vi "Loop.vi"(8 "error in":errorcluster, 10 "UI Queue":refnum<queue>, 11 "Controller Queue":T1) -> (0 "error out":errorcluster)   [LabVIEW 2019, in "Controller.lvlib"]
uses:
  Controller.lvlib
  UI/Update Message.ctl
  UI/Update Command.ctl
  Controller Message Queue.ctl
  Controller Message.ctl
  MDS Command.ctl
  Controller States.ctl
  Serial Info.ctl
  VMode.ctl
  IMode.ctl
  <vilib>/Instr/_visa.llb/VISA Configure Serial Port (Instr).vi
  UI/UI.lvlib
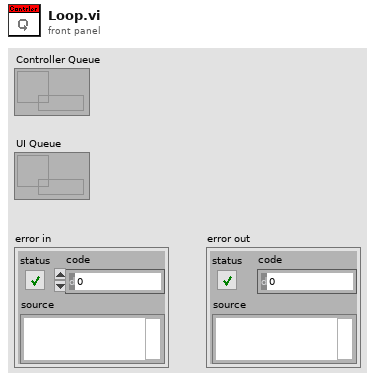
[diagram p1: front panel]
types:
  T1 = typedef "Controller.lvlib/Controller Message Queue.ctl" = refnum<queue>
  T2 = typedef "Controller.lvlib/Controller Message.ctl" = cluster{"MDS Command":T3, "Channel":u8, "Value":variant}
  T3 = typedef "Controller.lvlib/MDS Command.ctl" = enum16{"Idle", "Open", "Set VMode", "Set IMode", "Get Frequency", "Set Frequency", "Get Power", "Set Power (dBm)", "Set Power (%)", "Get Switch", "Switch Channel", "Store", "Wait for Prompt", "Wait for State", "Reset", "Error", "Close", "Stop"}
  T4 = typedef "Controller.lvlib/Controller States.ctl" = cluster{"Resource":refnum<visa-resource-name>}
  T5 = typedef "Controller.lvlib/Serial Info.ctl" = cluster{"Port":refnum<visa-resource-name>, "Baud Rate":u32}
  T6 = typedef "Controller.lvlib/VMode.ctl" = enum8{"5V", "10V"}
  T7 = typedef "Controller.lvlib/IMode.ctl" = enum8{"Internal", "External"}
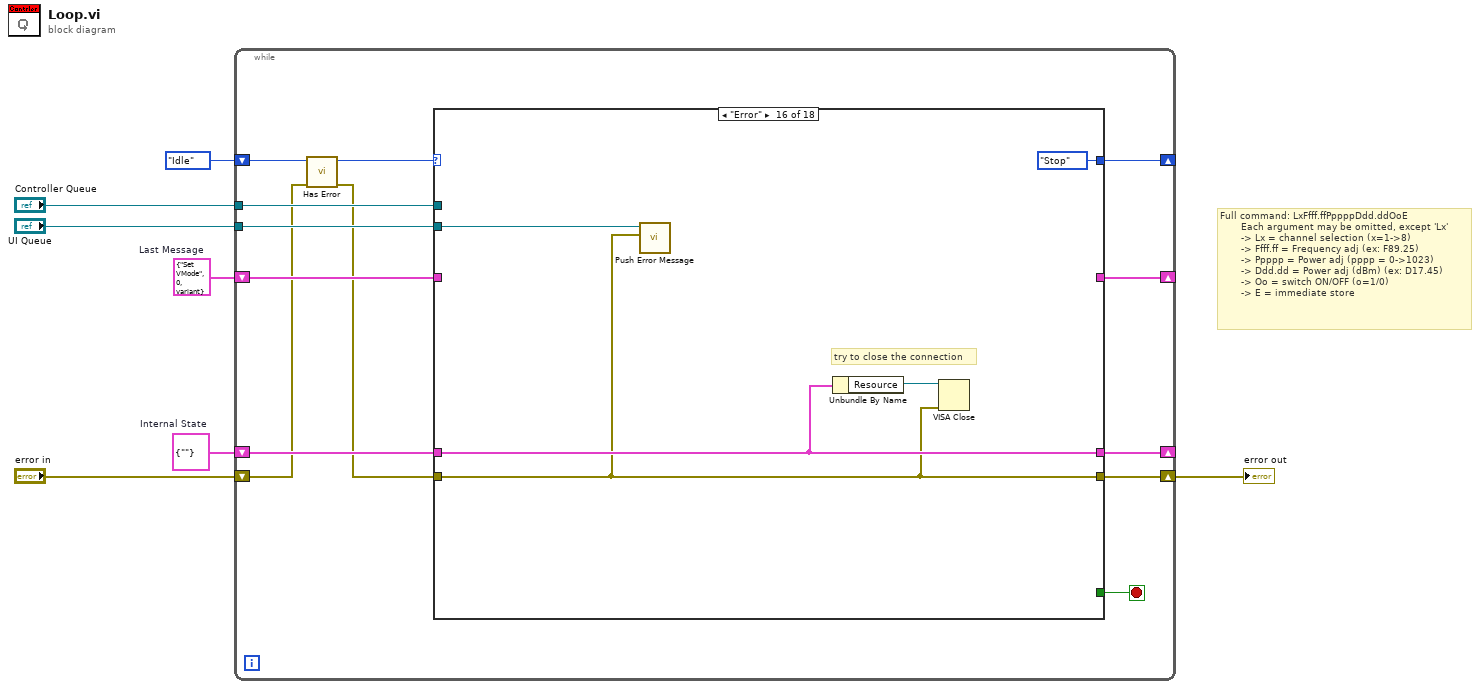
[diagram p0: block diagram]
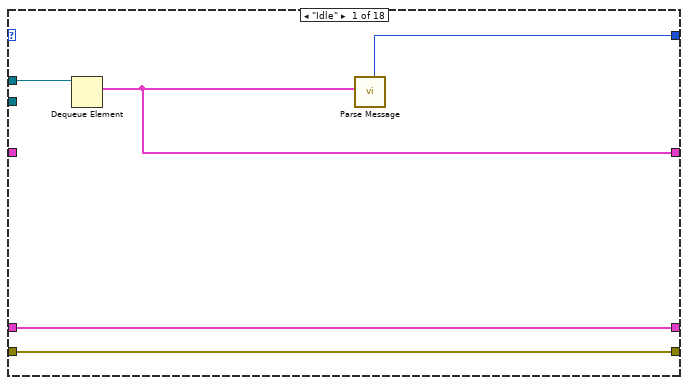
[diagram p2: hidden frame]
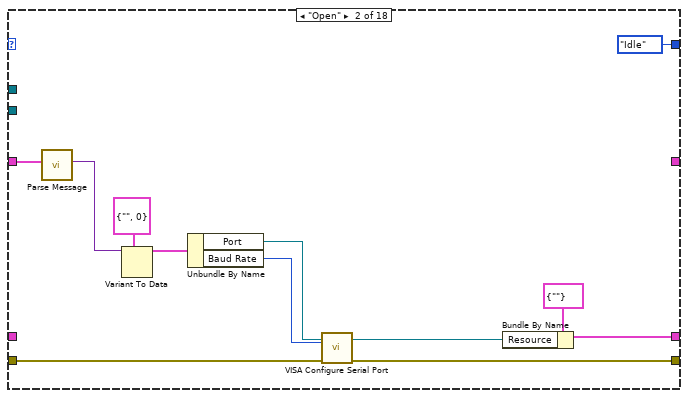
[diagram p3: hidden frame]
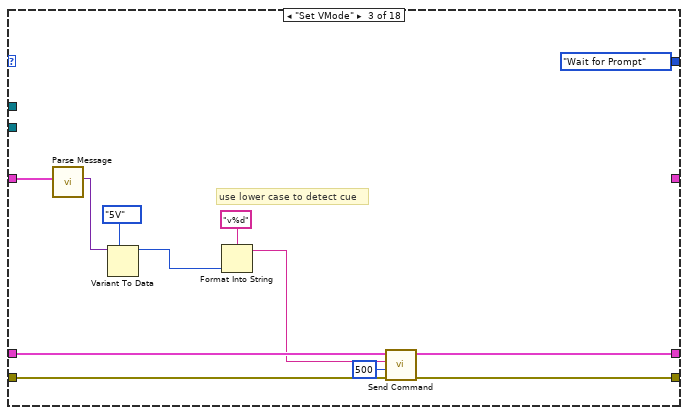
[diagram p4: hidden frame]
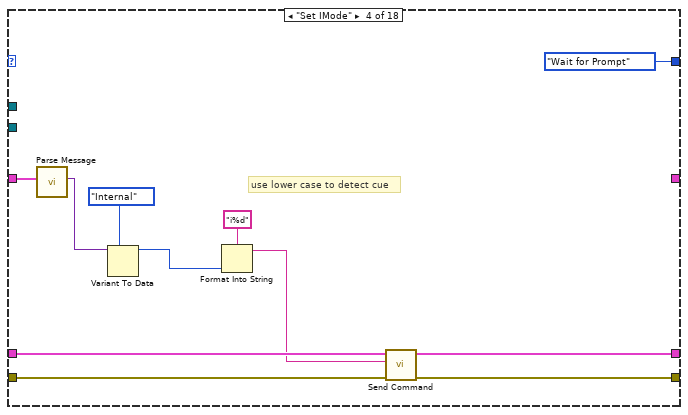
[diagram p5: hidden frame]
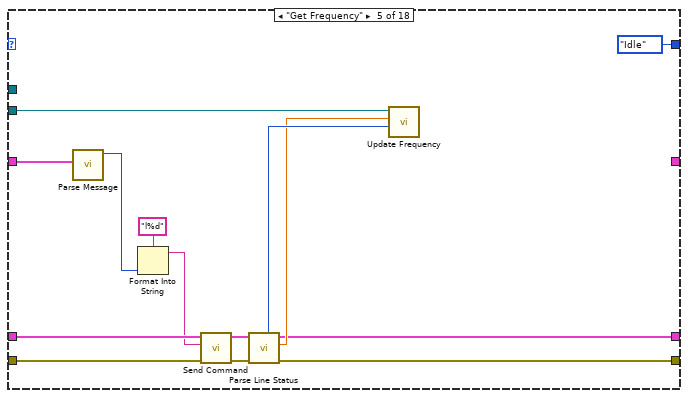
[diagram p6: hidden frame]
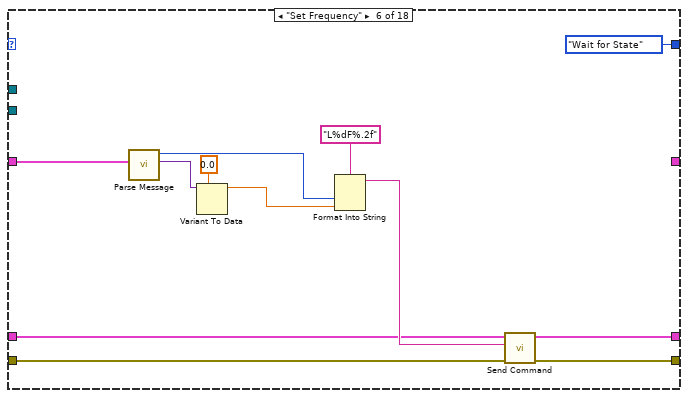
[diagram p7: hidden frame]
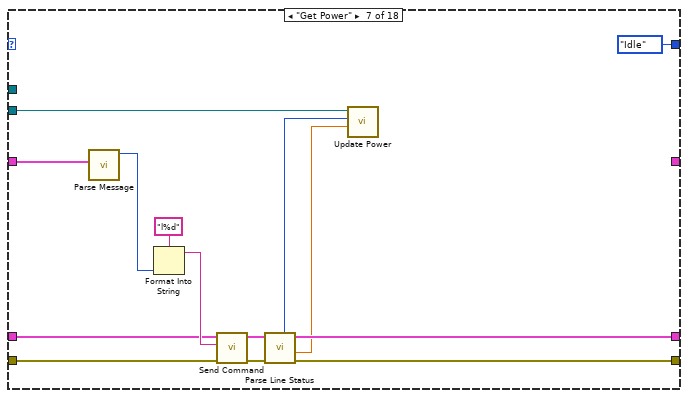
[diagram p8: hidden frame]
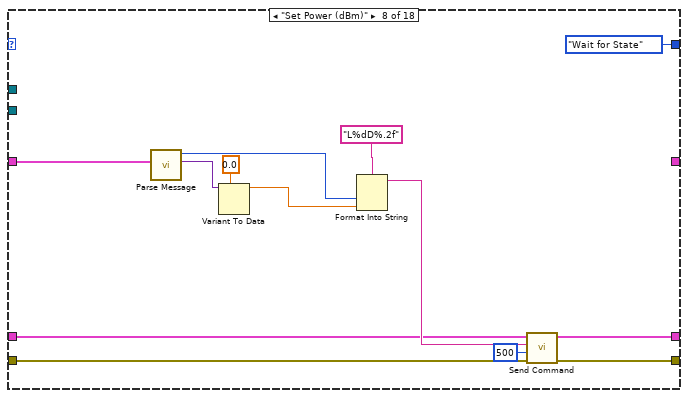
[diagram p9: hidden frame]
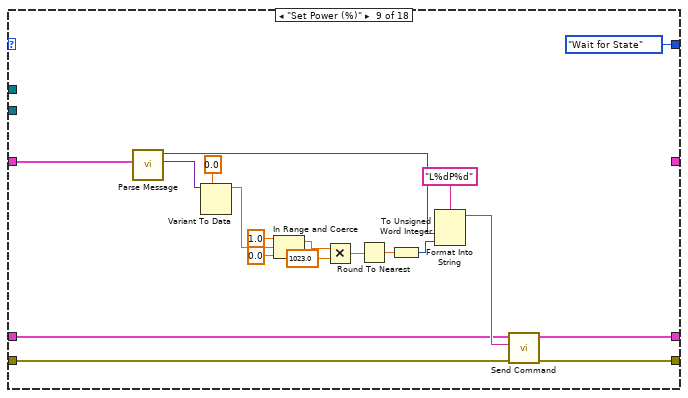
[diagram p10: hidden frame]
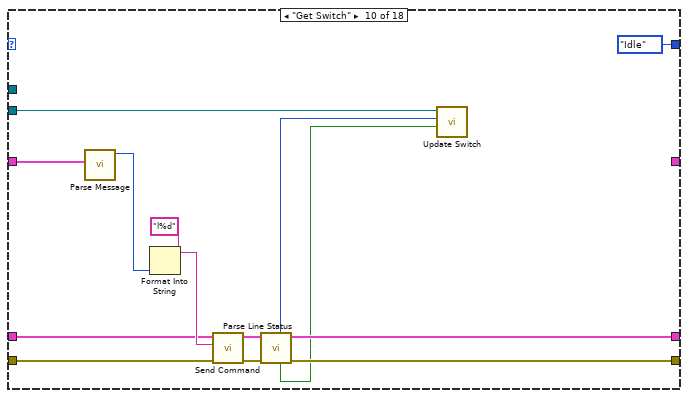
[diagram p11: hidden frame]
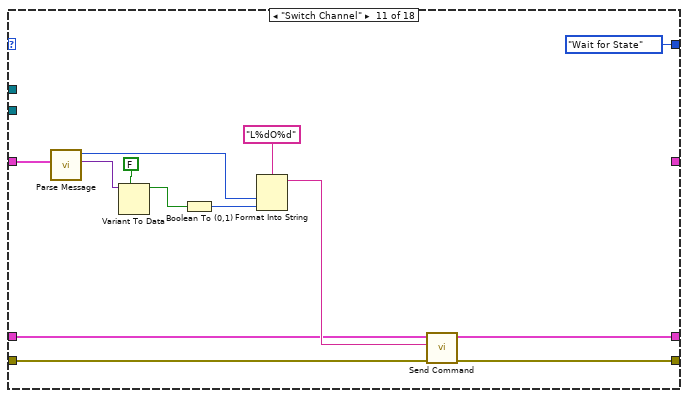
[diagram p12: hidden frame]
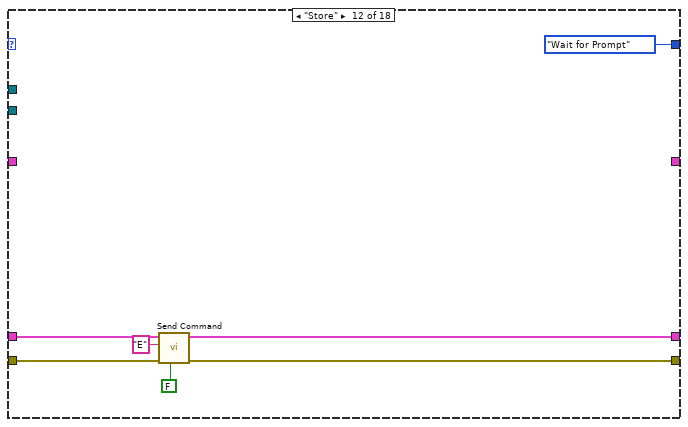
[diagram p13: hidden frame]
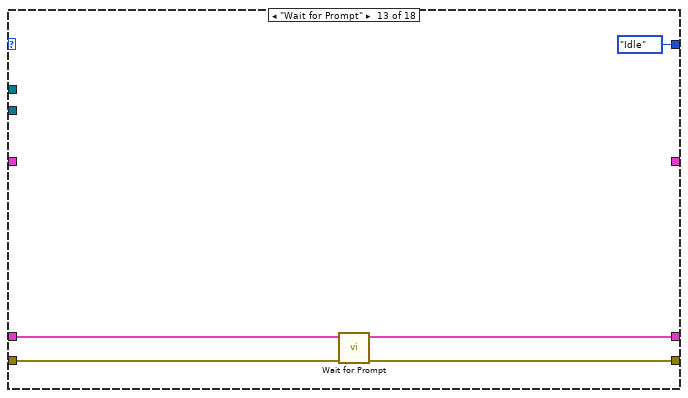
[diagram p14: hidden frame]
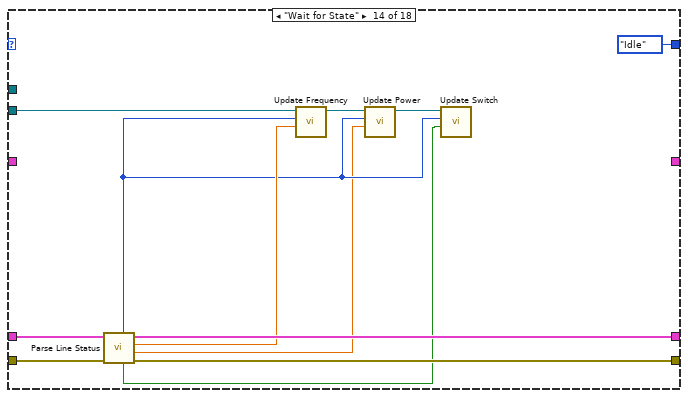
[diagram p15: hidden frame]
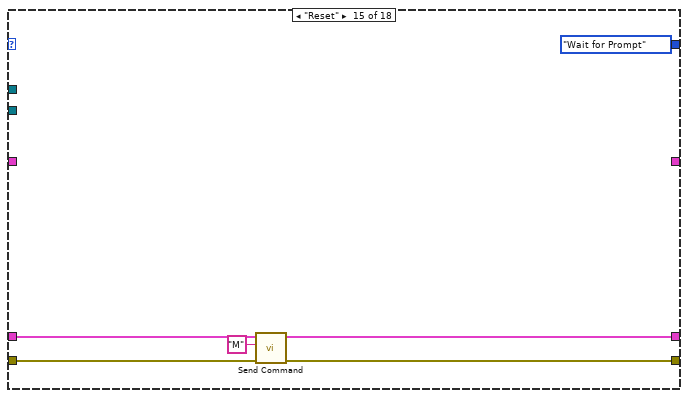
[diagram p16: hidden frame]
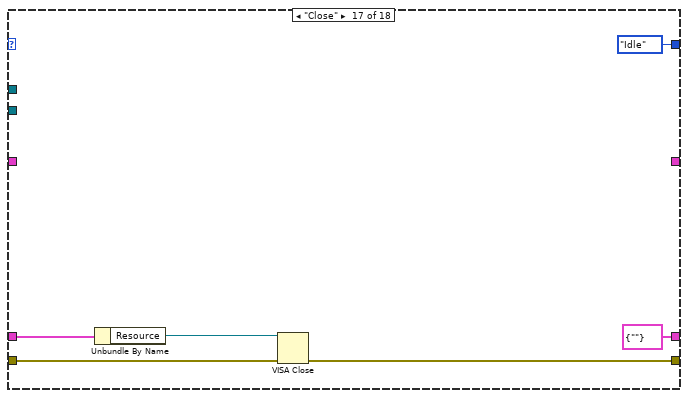
[diagram p17: hidden frame]
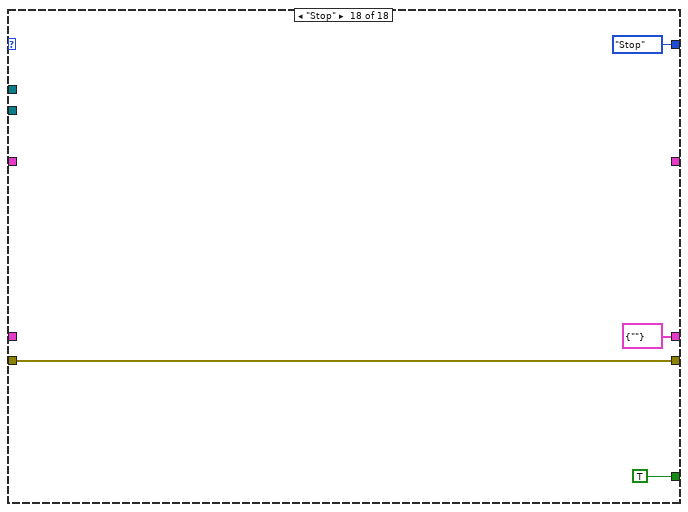
[diagram p18: hidden frame]
diagram:
  w5 = T2 {"MDS Command"=enum."Set VMode", "Channel"=0, "Value"=variant}  # Last Message
  w7 = T4 {"Resource"=""}  # Internal State
  # "Full command: LxFfff.ffPppppDdd.ddOoE\n       Each argument may be omitted, except 'Lx'\n       -> Lx = channel selection (x=1->8)\n       -> Ffff.ff = Frequency adj (ex: F89.25)\n       -> Ppppp = Power adj (pppp = 0->1023)\n       -> Ddd.dd = Power adj (dBm) (ex: D17.45)\n       -> Oo = switch ON/OFF (o=1/0)\n       -> E = immediate store"
  n1 = while {
    tunnel: "Controller Queue" -> [w17]
    shift-right: [w20] -> _
    shift-left: w7 -> [w19]
    shift-right: [w14] -> w4
    shift-left: "error in" -> [w8]
    shift-right: [w15] -> _
    shift-left: w5 -> [w16]
    shift-right: [w12] -> _
    shift-left: MDS_Command."Idle" ("MDS Command") -> [w11]
    tunnel: "UI Queue" -> [w13]
    stop <- w18 stop-if-true
    n2 = call "Has Error.vi"("error in (no error)"=w8, "MDS Command in"=w11) -> ("error out"=w9:errorcluster, "MDS Command out"=w10:T3)  [unwired: 8 in]
    n3 = case shown="\"Error\"" w10 {
      tunnel: [w25 w33 w39 w50 w70 w79 w92 w103 w122 w138 w147 w161 w167 w180 w184 w193 T4 {"Resource"=""} T4 {"Resource"=""}] -> w20
      tunnel: w19 -> [w25 _ w47 w57 w67 w81 w93 w106 w126 w141 w150 w166 w170 w182 w187 w193 w199 _]
      tunnel: w9 -> [w24 w30 w48 w59 w68 w80 w94 w105 w125 w140 w149 w165 w169 w181 w186 w190 w197 w204]
      tunnel: [w24 w29 w38 w58 w71 w78 w91 w104 w123 w139 w148 w160 w168 w179 w185 w190 w196 w204] -> w14
      tunnel: [_ _ _ _ _ _ _ _ _ _ _ _ _ _ _ _ _ TRUE] -> w18
      tunnel: w17 -> [w23 _ _ _ _ _ _ _ _ _ _ _ _ _ _ _ _ _]
      tunnel: w16 -> [_ w27 w41 w52 w63 w77 w90 w102 w124 w136 w158 _ _ _ _ _ _ _]
      tunnel: [w22 _ _ _ _ _ _ _ _ _ _ _ _ _ _ _ _ _] -> w15
      tunnel: [w21 MDS_Command."Idle" ("MDS Command") MDS_Command."Wait for Prompt" ("MDS Command") MDS_Command."Wait for Prompt" ("MDS Command") MDS_Command."Idle" ("MDS Command") MDS_Command."Wait for State" ("MDS Command") MDS_Command."Idle" ("MDS Command") MDS_Command."Wait for State" ("MDS Command") MDS_Command."Wait for State" ("MDS Command") MDS_Command."Idle" ("MDS Command") MDS_Command."Wait for State" ("MDS Command") MDS_Command."Wait for Prompt" ("MDS Command") MDS_Command."Idle" ("MDS Command") MDS_Command."Idle" ("MDS Command") MDS_Command."Wait for Prompt" ("MDS Command") MDS_Command."Stop" ("MDS Command") MDS_Command."Idle" ("MDS Command") MDS_Command."Stop" ("MDS Command")] -> w12
      tunnel: w13 -> [_ _ _ _ w69 _ w89 _ _ w135 _ _ _ w178 _ w191 _ _]
      frame "Idle" {
        n4 = Dequeue Element(queue=w23) -> (element=w22:T2)  [unwired: 2 in, 3 out]
        n5 = call "Parse Message.vi"("Controller Message"=w22) -> ("MDS Command"=w21:T3)  [unwired: 7 in, 2 out]
      }
      frame "Open" {
        n6 = call "Parse Message.vi"("Controller Message"=w27) -> ("Value"=w26:variant)  [unwired: 7 in, 2 out]
        n7 = Variant To Data(type=T5 {"Port"="", "Baud Rate"=0} ("Serial Info"), Variant=w26) -> (data=w36:T5)  [unwired: 1 in, 1 out]
        n8 = Unbundle By Name(w36) -> ("Port"=w35:refnum<visa-resource-name>, "Baud Rate"=w34:u32)
        n9 = call-poly "VISA Configure Serial Port"("VISA resource name"=w35, "baud rate (9600)"=w34, "error in (no error)"=w30) -> ("VISA resource name out"=w31:refnum<visa-resource-name>, "error out"=w29:errorcluster)  [unwired: 11 in]
        n10 = Bundle By Name(cluster=T4 {"Resource"=""}, "Resource"=w31) -> (w33:T4)
      }
      frame "Set VMode" {
        # "use lower case to detect cue"
        n11 = call "Parse Message.vi"("Controller Message"=w41) -> ("Value"=w40:variant)  [unwired: 7 in, 2 out]
        n12 = Variant To Data(type=VMode."5V" ("VMode"), Variant=w40) -> (data=w43:T6)  [unwired: 1 in, 1 out]
        n13 = Format Into String(format string="v%d", w43) -> (resulting string=w46:string)  [unwired: 2 in, 1 out]
        n14 = call "Send Command.vi"("error in (no error)"=w48, "Delay (ms)"=u32 500, "Command"=w46, "Controller States in"=w47) -> ("error out"=w38:errorcluster, "Controller States out"=w39:T4)  [unwired: 6 in]
      }
      frame "Set IMode" {
        # "use lower case to detect cue"
        n15 = call "Parse Message.vi"("Controller Message"=w52) -> ("Value"=w51:variant)  [unwired: 7 in, 2 out]
        n16 = Variant To Data(type=IMode."Internal" ("IMode"), Variant=w51) -> (data=w55:T7)  [unwired: 1 in, 1 out]
        n17 = Format Into String(format string="i%d", w55) -> (resulting string=w56:string)  [unwired: 2 in, 1 out]
        n18 = call "Send Command.vi"("error in (no error)"=w59, "Command"=w56, "Controller States in"=w57) -> ("error out"=w58:errorcluster, "Controller States out"=w50:T4)  [unwired: 7 in]
      }
      frame "Get Frequency" {
        n19 = call "Parse Message.vi"("Controller Message"=w63) -> ("Channel"=w62:u8)  [unwired: 7 in, 2 out]
        n20 = Format Into String(format string="l%d", w62) -> (resulting string=w61:string)  [unwired: 2 in, 1 out]
        n21 = call "Send Command.vi"("error in (no error)"=w68, "Command"=w61, "Controller States in"=w67) -> ("error out"=w65:errorcluster, "Controller States out"=w66:T4)  [unwired: 7 in]
        n22 = call "Parse Line Status.vi"("error in (no error)"=w65, "Controller States in"=w66) -> ("error out"=w71:errorcluster, "Frequency (MHz)"=w72:dbl, "Controller States out"=w70:T4, "Channel"=w73:u8)  [unwired: 4 in, 2 out]
        n23 = call "Update Frequency.vi"("Frequency (MHz)"=w73, "Channel"=w72, "UI Queue in"=w69) -> ()  [unwired: 8 in, 1 out]
      }
      frame "Set Frequency" {
        n24 = call "Parse Message.vi"("Controller Message"=w77) -> ("Channel"=w83:u8, "Value"=w82:variant)  [unwired: 7 in, 1 out]
        n25 = Variant To Data(type=0.0, Variant=w82) -> (data=w75:dbl)  [unwired: 1 in, 1 out]
        n26 = Format Into String(format string="L%dF%.2f", w83, w75) -> (resulting string=w84:string)  [unwired: 2 in, 1 out]
        n27 = call "Send Command.vi"("error in (no error)"=w80, "Command"=w84, "Controller States in"=w81) -> ("error out"=w78:errorcluster, "Controller States out"=w79:T4)  [unwired: 7 in]
      }
      frame "Get Power" {
        n28 = call "Parse Message.vi"("Controller Message"=w90) -> ("Channel"=w96:u8)  [unwired: 7 in, 2 out]
        n29 = Format Into String(format string="l%d", w96) -> (resulting string=w95:string)  [unwired: 2 in, 1 out]
        n30 = call "Send Command.vi"("error in (no error)"=w94, "Command"=w95, "Controller States in"=w93) -> ("error out"=w98:errorcluster, "Controller States out"=w99:T4)  [unwired: 7 in]
        n31 = call "Parse Line Status.vi"("error in (no error)"=w98, "Controller States in"=w99) -> ("error out"=w91:errorcluster, "Power (dBm)"=w88:dbl, "Controller States out"=w92:T4, "Channel"=w87:u8)  [unwired: 4 in, 2 out]
        n32 = call "Update Power.vi"("Power (dBm)"=w88, "Channel"=w87, "UI Queue in"=w89) -> ()  [unwired: 8 in, 1 out]
      }
      frame "Set Power (dBm)" {
        n33 = call "Parse Message.vi"("Controller Message"=w102) -> ("Channel"=w110:u8, "Value"=w109:variant)  [unwired: 7 in, 1 out]
        n34 = Variant To Data(type=0.0, Variant=w109) -> (data=w107:dbl)  [unwired: 1 in, 1 out]
        n35 = Format Into String(format string="L%dD%.2f", w110, w107) -> (resulting string=w111:string)  [unwired: 2 in, 1 out]
        n36 = call "Send Command.vi"("error in (no error)"=w105, "Delay (ms)"=u32 500, "Command"=w111, "Controller States in"=w106) -> ("error out"=w104:errorcluster, "Controller States out"=w103:T4)  [unwired: 6 in]
      }
      frame "Set Power (%)" {
        n37 = call "Parse Message.vi"("Controller Message"=w124) -> ("Channel"=w129:u8, "Value"=w128:variant)  [unwired: 7 in, 1 out]
        n38 = Variant To Data(type=0.0, Variant=w128) -> (data=w119:dbl)  [unwired: 1 in, 1 out]
        n39 = In Range and Coerce(upper limit=1.0, x=w119, lower limit=0.0) -> (coerced(x)=w118:dbl)  [unwired: 1 out]
        n40 = Multiply(x=w118, y=1023.0) -> (x*y=w116:dbl)
        n41 = Round To Nearest(number=w116) -> (nearest integer value=w115:dbl)
        n42 = To Unsigned Word Integer(number=w115) -> (unsigned 16bit integer=w114:u16)
        n43 = Format Into String(format string="L%dP%d", w129, w114) -> (resulting string=w130:string)  [unwired: 2 in, 1 out]
        n44 = call "Send Command.vi"("error in (no error)"=w125, "Command"=w130, "Controller States in"=w126) -> ("error out"=w123:errorcluster, "Controller States out"=w122:T4)  [unwired: 7 in]
      }
      frame "Get Switch" {
        n45 = call "Parse Message.vi"("Controller Message"=w136) -> ("Channel"=w145:u8)  [unwired: 7 in, 2 out]
        n46 = Format Into String(format string="l%d", w145) -> (resulting string=w146:string)  [unwired: 2 in, 1 out]
        n47 = call "Send Command.vi"("error in (no error)"=w140, "Command"=w146, "Controller States in"=w141) -> ("error out"=w144:errorcluster, "Controller States out"=w143:T4)  [unwired: 7 in]
        n48 = call "Parse Line Status.vi"("error in (no error)"=w144, "Controller States in"=w143) -> ("error out"=w139:errorcluster, "Controller States out"=w138:T4, "Switch"=w133:bool, "Channel"=w134:u8)  [unwired: 4 in, 2 out]
        n49 = call "Update Switch.vi"("On/Off"=w133, "Channel"=w134, "UI Queue in"=w135) -> ()  [unwired: 8 in, 1 out]
      }
      frame "Switch Channel" {
        n50 = call "Parse Message.vi"("Controller Message"=w158) -> ("Channel"=w155:u8, "Value"=w154:variant)  [unwired: 7 in, 1 out]
        n51 = Variant To Data(type=FALSE, Variant=w154) -> (data=w152:bool)  [unwired: 1 in, 1 out]
        n52 = Boolean To (0,1)(Boolean=w152) -> (0, 1=w151:i16)
        n53 = Format Into String(format string="L%dO%d", w155, w151) -> (resulting string=w156:string)  [unwired: 2 in, 1 out]
        n54 = call "Send Command.vi"("error in (no error)"=w149, "Command"=w156, "Controller States in"=w150) -> ("error out"=w148:errorcluster, "Controller States out"=w147:T4)  [unwired: 7 in]
      }
      frame "Store" {
        n55 = call "Send Command.vi"("Line Break (T)?"=FALSE, "error in (no error)"=w165, "Command"="E", "Controller States in"=w166) -> ("error out"=w160:errorcluster, "Controller States out"=w161:T4)  [unwired: 6 in]
      }
      frame "Wait for Prompt" {
        n56 = call "Wait for Prompt.vi"("error in (no error)"=w169, "Controller States in"=w170) -> ("error out"=w168:errorcluster, "Controller States out"=w167:T4)  [unwired: 7 in, 1 out]
      }
      frame "Wait for State" {
        n57 = call "Parse Line Status.vi"("error in (no error)"=w181, "Controller States in"=w182) -> ("error out"=w179:errorcluster, "Power (dBm)"=w173:dbl, "Frequency (MHz)"=w177:dbl, "Controller States out"=w180:T4, "Switch"=w172:bool, "Channel"=w174:u8)  [unwired: 4 in]
        n58 = call "Update Frequency.vi"("Frequency (MHz)"=w177, "Channel"=w174, "UI Queue in"=w178) -> ("UI Queue out"=w176:refnum<queue>)  [unwired: 8 in]
        n59 = call "Update Power.vi"("Power (dBm)"=w173, "Channel"=w174, "UI Queue in"=w176) -> ("UI Queue out"=w175:refnum<queue>)  [unwired: 8 in]
        n60 = call "Update Switch.vi"("On/Off"=w172, "Channel"=w174, "UI Queue in"=w175) -> ()  [unwired: 8 in, 1 out]
      }
      frame "Reset" {
        n61 = call "Send Command.vi"("error in (no error)"=w186, "Command"="M", "Controller States in"=w187) -> ("error out"=w185:errorcluster, "Controller States out"=w184:T4)  [unwired: 7 in]
      }
      frame "Error" {
        # "try to close the connection"
        n62 = call "Push Error Message.vi"("error constant"=w190, "UI Queue in"=w191) -> ()  [unwired: 9 in, 1 out]
        n63 = Unbundle By Name(w193) -> ("Resource"=w192:refnum<visa-resource-name>)
        n64 = VISA Close(VISA resource name=w192, error in (no error)=w190) -> ()  [unwired: 1 out]
      }
      frame "Close" {
        n65 = Unbundle By Name(w199) -> ("Resource"=w198:refnum<visa-resource-name>)
        n66 = VISA Close(VISA resource name=w198, error in (no error)=w197) -> (error out=w196:errorcluster)
      }
      frame "Stop" {
      }
    }
  }
  "error out" <- w4
